vi "fpga_Fund LP2 Filter Parallel Path.vi"(0 "re":fxp<+/-,32,5>, 1 "reset":bool, 5 "im":fxp<+/-,32,5>, 7 "#Ch":fxp<+,5,5>=16.0, 9 "input valid":bool) -> (4 "re filtered":fxp<+/-,32,6>, 6 "im filtered":fxp<+/-,32,6>, 10 "output valid":bool, 14 "ready for input":bool)   [LabVIEW 2012, in "NI_EP_Protection_FPGA.lvlib"]
doc: "----------------------\n\nThis filter is configured as follows:\n\n<b>Filter Configuration</b>\nType: Single Rate\nStructure: FIR Direct Form\n\n<b>Input Data Type</b>\nType: fixed-point <±,32,5> [-1.600000E+1,1.600000E+1]:7.450581E-9\n\n<b>Output Data Type</b>\nType: fixed-point <±,32,6> [-3.200000E+1,3.200000E+1]:1.490116E-8\nRounding mode: Truncate\nOverflow mode: Wrap\n\n<b>Implementation</b>\nNumber of channels: 16\nMaximum input sampling rate per channel @ 40MHz: 55.556kHz\nGain processing: On Host\nMethod: Multiply-Accumulate\nNumber of parallel data path: 2\nTotal number of channels: 32\nNumber of multiply pipeline stages: 1\nMultiply register in: False\nNumber of adder levels per register: 2\nState memory: Block Memory\nCoefficient memory: ROM\n\n<b>Execution Mode</b>\nInside single-cycle Timed Loop\nThroughput: 45 cycles/sample\n\n<b>Estimated Resources</b>\nTotal number of multiply-accumulate units: 2\nNumber of multiply-accumulate units per data path: 1\nMultiply operation: I32.5 x I17.-3 => I32.6"
uses:
  <vilib>/addons/Electrical Power/Protection/NI_EP_Protection_FPGA.lvlib
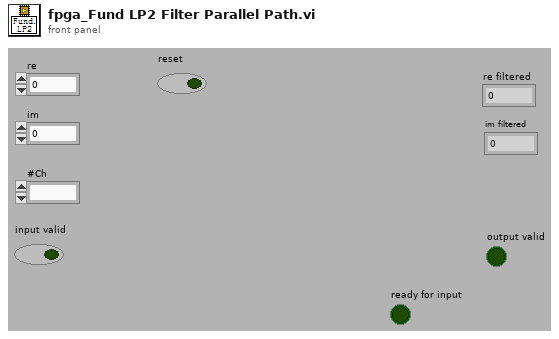
[diagram p1: front panel]
types:
  T1 = cluster{"WREn":bool, "WRAddr":fxp<+,10,10>, "RDAddr":fxp<+,10,10>, "BufWREn":bool, "BufWRAddr":fxp<+,10,10>, "firstRun":bool, "BufFiirstRun":bool}
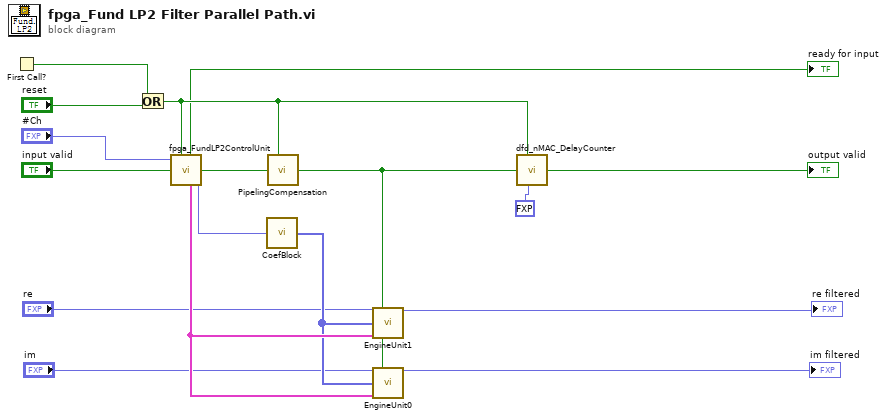
[diagram p0: block diagram]
diagram:
  n1 = First Call?() -> (First Call?: T/F=w14:bool)
  n2 = Or(x=w14, y="reset") -> (x .or. y?=w13:bool)
  n3 = call <vilib>:"fpga_FundLP2ControlUnit.vi"("#Ch"="#Ch", "reset"=w13, "input valid"="input valid") -> ("ready for input"=→"ready for input":bool, "output valid"=w16:bool, "opState"=w10:T1, "coefRDAddr"=w11:fxp<+,6,6>)  [unwired: 3 in]
  n4 = call "CoefBlock"("coefAddr"=w11) -> ("coefficients"=w7:fxp<+/-,17,-3>[])  [unwired: 8 in]
  n5 = call "PipelingCompensation"("reset"=w13, "data in"=w16) -> ("data out"=w9:bool)  [unwired: 7 in]
  n6 = call "EngineUnit1"("input data"="re", "ACC_Load"=w9, "coefficients"=w7, "opState"=w10) -> ("output data"=→"re filtered":fxp<+/-,32,6>)  [unwired: 11 in]
  n7 = call "EngineUnit0"("input data"="im", "ACC_Load"=w9, "coefficients"=w7, "opState"=w10) -> ("output data"=→"im filtered":fxp<+/-,32,6>)  [unwired: 11 in]
  n8 = call "dfd_nMAC_DelayCounter.vi"("reset"=w13, "data in"=w9, "#delay"=fxp<+,6,6> 45.0 ("#TPPM")) -> ("data out"=→"output valid":bool)  [unwired: 6 in]
